vi "Multidimensional Test Function.vi"(1 "(x_1,...,x_n)":refnum<class "Dual.lvclass">[](array[class])) -> (0 "f(x_1,...,x_n)":refnum<class "Dual.lvclass">)   [LabVIEW 2020, in "Tests.lvlib"]
uses:
  Tests.lvlib
  classes/Dual/Dual.lvclass
  classes/Dual/Dual.lvclass/Dual.ctl
  cbc49117-5460-4464-b1ce-91b60d1512c3.vi
  c79a468e-ecb6-4346-9dae-677225388434.vi
  7deeae57-a460-4186-b5c0-7bfd187d755c.vi
  91b2807f-5384-433c-98fd-9cb31c3ad06d.vi
  48db8747-0669-4619-97c1-2a1e713ea16f.vi
  93f81844-541a-49dd-9aca-1117755405ff.vi
  cbc49117-5460-4464-b1ce-91b60d1512c3.vi/957074e8-cc3b-4647-8ff1-d975a744cd4e.vi
  classes/Dual/Write a and b.vi
  classes/Dual/Read a and b.vi
  c79a468e-ecb6-4346-9dae-677225388434.vi/957074e8-cc3b-4647-8ff1-d975a744cd4e.vi
  7deeae57-a460-4186-b5c0-7bfd187d755c.vi/b6499733-2759-4852-aa6b-3ec1516ef704.vi
  7deeae57-a460-4186-b5c0-7bfd187d755c.vi/ce7907ec-4dc6-4618-8708-ad667a8e3a23.vi
  91b2807f-5384-433c-98fd-9cb31c3ad06d.vi/cbb88b8f-dcf9-42b8-ac98-84298073c153.vi
  48db8747-0669-4619-97c1-2a1e713ea16f.vi/6101d903-ff9f-41ff-96b8-b42400c258cc.vi
  48db8747-0669-4619-97c1-2a1e713ea16f.vi/5aba97ba-e1f8-4e08-94e3-f0ae7cb31178.vi
  93f81844-541a-49dd-9aca-1117755405ff.vi/6101d903-ff9f-41ff-96b8-b42400c258cc.vi
  93f81844-541a-49dd-9aca-1117755405ff.vi/5aba97ba-e1f8-4e08-94e3-f0ae7cb31178.vi
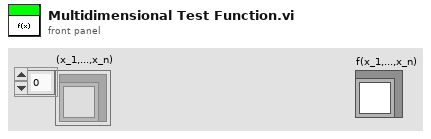
[diagram p1: front panel]
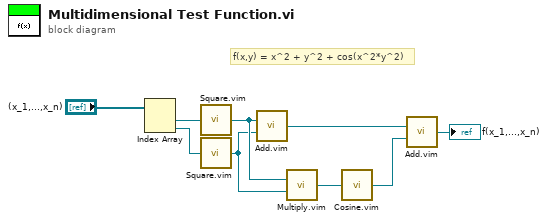
[diagram p0: block diagram]
diagram:
  # "f(x,y) = x^2 + y^2 + cos(x^2*y^2)"
  n1 = Index Array(array="(x_1,...,x_n)") -> (element #1=w8:refnum<class "Dual.lvclass">, element #2=w2:refnum<class "Dual.lvclass">)  [unwired: 2 in]
  n2 = call "Square.vim"("x"=w8) -> ("x^2"=w6:refnum<class "Dual.lvclass">)
  n3 = call "Square.vim"("x"=w2) -> ("x^2"=w5:refnum<class "Dual.lvclass">)
  n4 = call "Add.vim"("x"=w6, "y"=w5) -> ("x + y"=w3:refnum<class "Dual.lvclass">)  [unwired: 13 in]
  n5 = call "Multiply.vim"("x"=w6, "y"=w5) -> ("x * y"=w1:refnum<class "Dual.lvclass">)  [unwired: 13 in]
  n6 = call "Cosine.vim"("x"=w1) -> ("cos(x)"=w4:refnum<class "Dual.lvclass">)
  n7 = call "Add.vim"("x"=w3, "y"=w4) -> ("x + y"=→"f(x_1,...,x_n)":refnum<class "Dual.lvclass">)  [unwired: 13 in]
